vi "更新程序.vi"() -> ()   [LabVIEW 2016, in "自动更新.lvlib"]
uses:
  <vilib>/FTP/NI_FTP.lvlib
panel:
  out "FTP链接结束":bool
  out "updateconfiguration":T1
  out "软件版本 2":string caption="目标软件版本"
  out "软件版本":string caption="当前软件版本"
  out "下载的文件名":string
  out "目标文件夹名":string
  out "端口号":i32
  out "IP地址":string
  out "步骤":string
  out "枚举":T2(ring)
  in  "目标路径（使用对话框）":path
  out "下载保存目录":path
  out "更新进度":u8(slide) scale=0.0..100.0
  # "1.先下载更新-------2.关闭主应用-------3.替换应用--------4.打开主应用-----------5.关闭本程序"
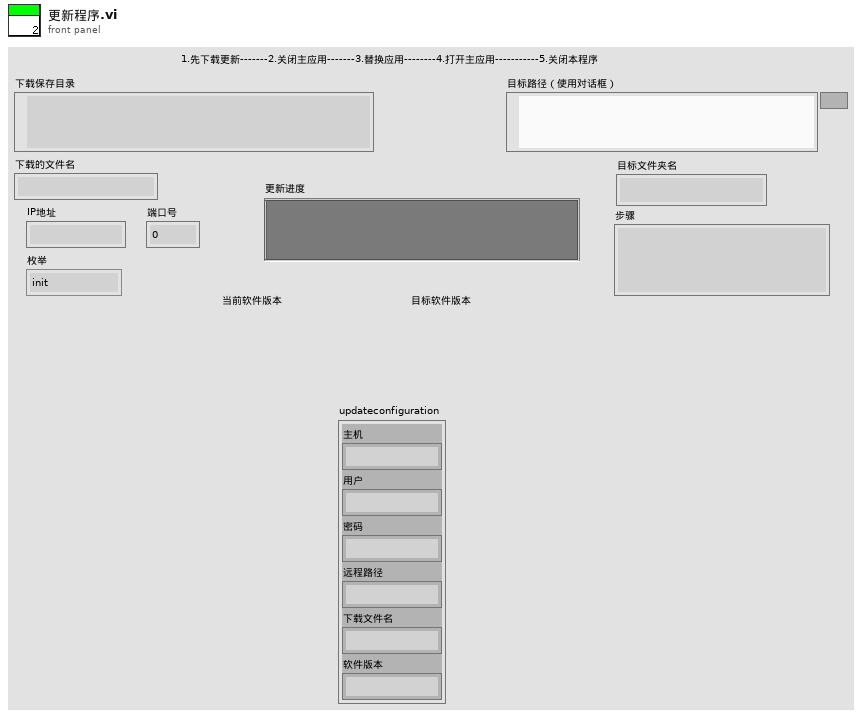
[diagram p1: front panel]
types:
  T1 = cluster{"主机":string, "用户":string, "密码":string, "远程路径":string, "下载文件名":string, "软件版本":string}
  T2 = enum16{"init", "download", "close", "replace", "open", "over"}
  T3 = typedef "NI_FTP.lvlib/FTP File Info.ctl" = cluster{"type":enum16{"unknown", "file", "dir", "link"}, "permissions":string, "owner":string, "group":string, "size":i32, "date":string, "name":string, "link name":string}
  T4 = enum16{"open", "replace", "create", "open or create", "replace or create", "replace or create with confirmation"}
  T5 = cluster{"网络灯":bool, "接收中":bool, "已接收百分比":u8, "接收成功次数":dbl, "当前步骤":enum16{"init", "receivehead", "receivecontent", "receivesuccess", "over"}, "文件名":string, "error out":errorcluster}
  T6 = cluster{"remote path":string, "local path":path, "binary":bool}
  T7 = typedef "NI_FTP.lvlib/FTP Session.ctl" = refnum<k5>
  T8 = cluster{"remote path":string, "local path":path, "binary":bool}[]
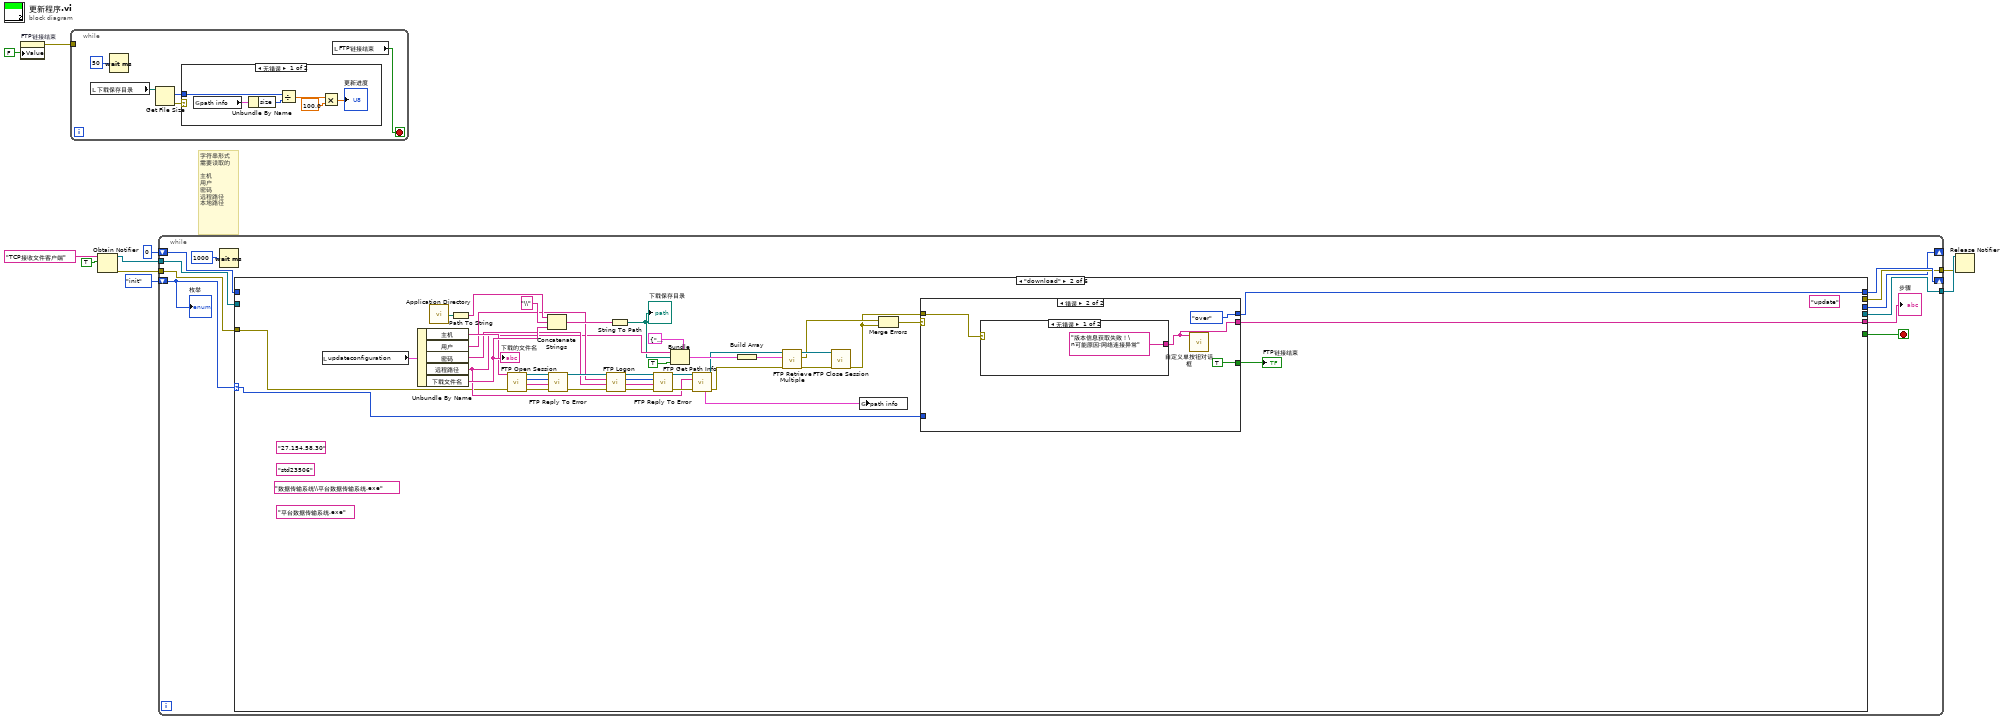
[diagram p0: block diagram]
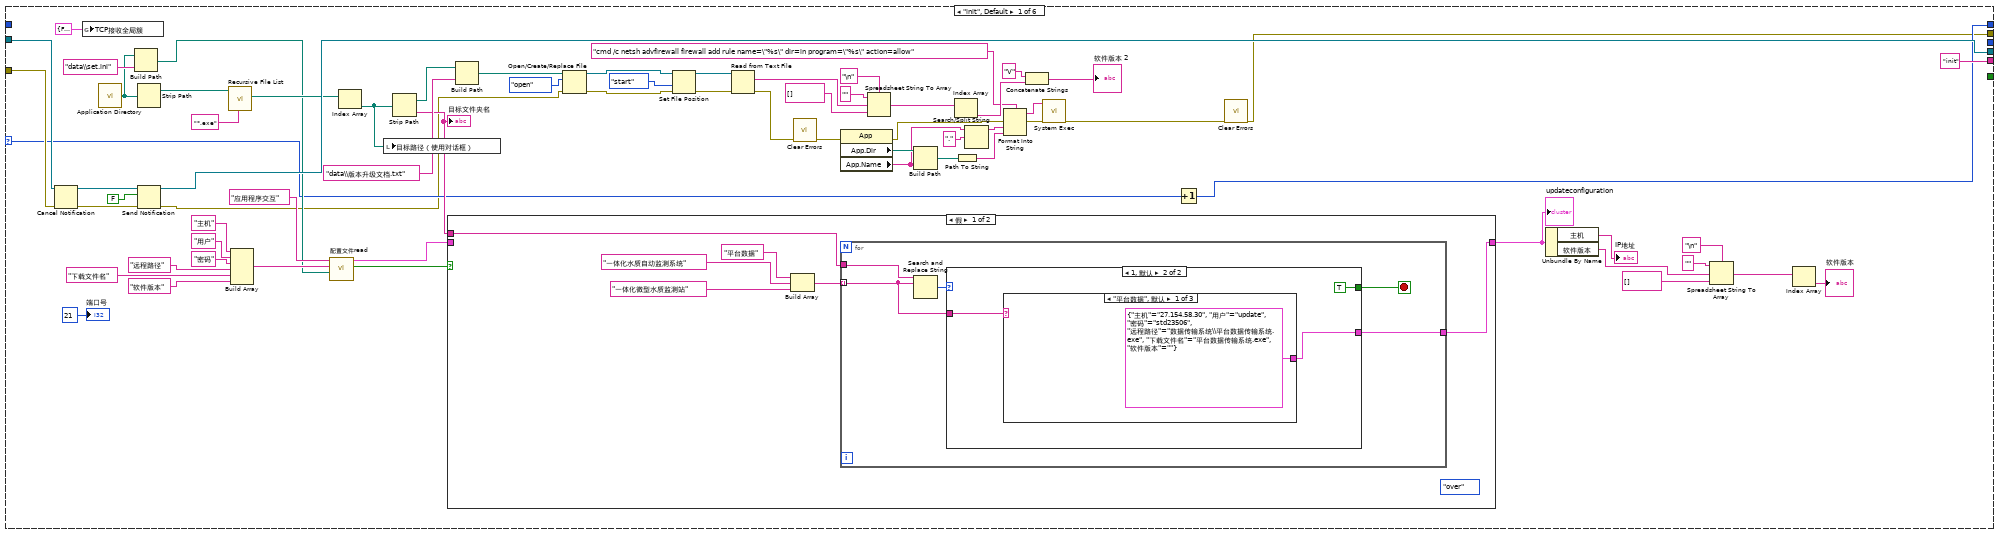
[diagram p3: hidden frame]
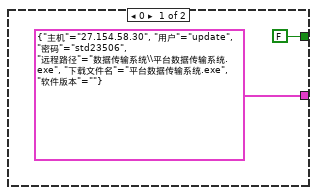
[diagram p4: hidden frame]
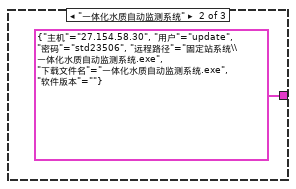
[diagram p5: hidden frame]
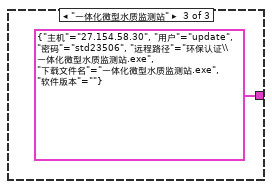
[diagram p6: hidden frame]
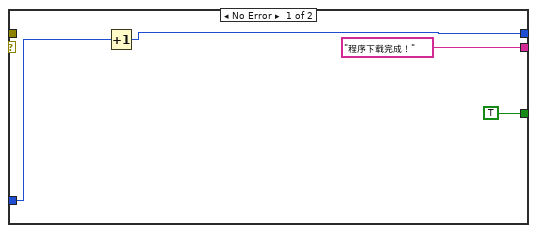
[diagram p8: hidden frame]
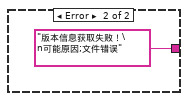
[diagram p9: hidden frame]
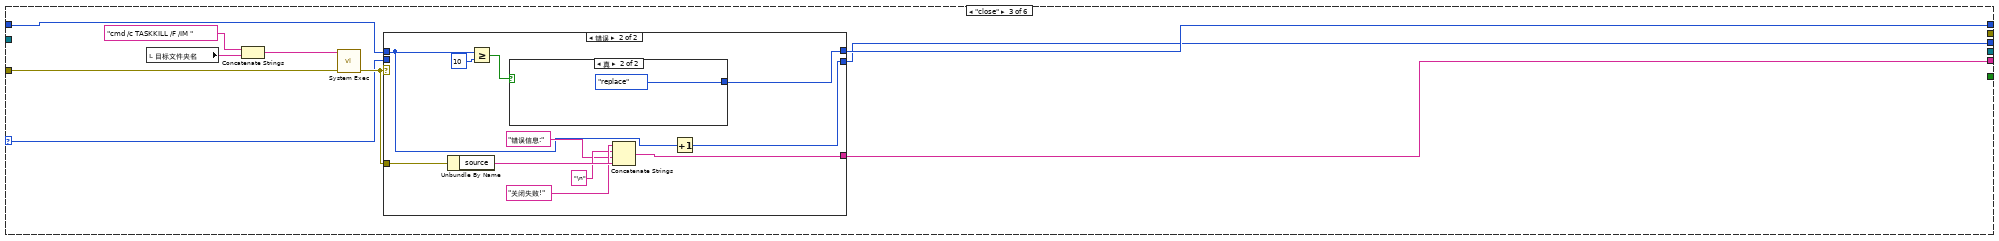
[diagram p10: hidden frame]
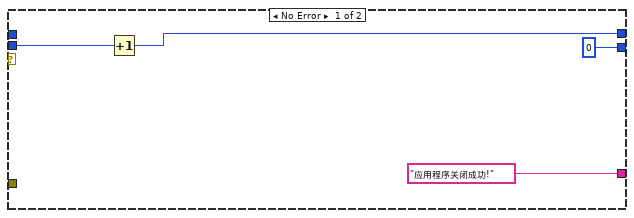
[diagram p11: hidden frame]
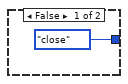
[diagram p12: hidden frame]
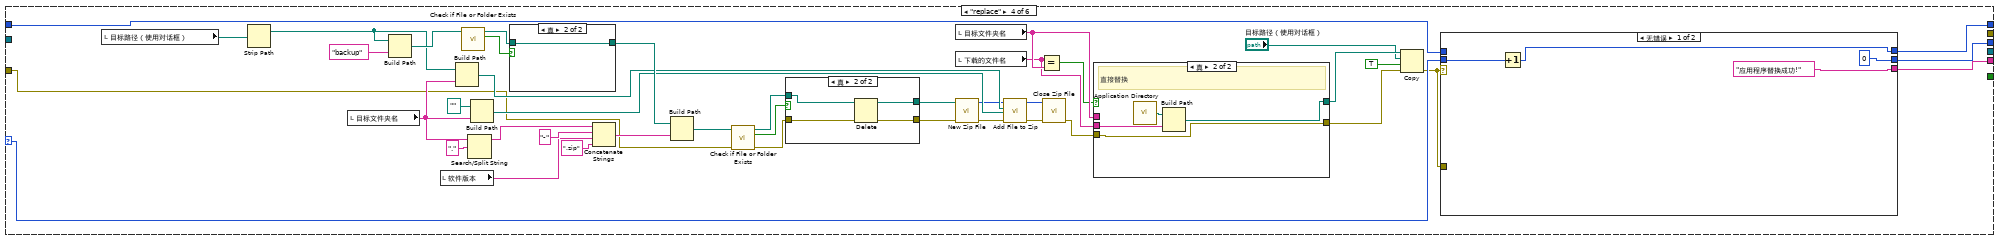
[diagram p13: hidden frame]
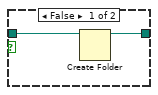
[diagram p15: hidden frame]
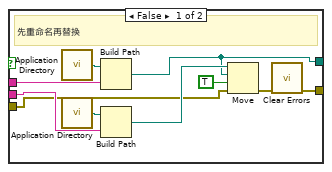
[diagram p16: hidden frame]
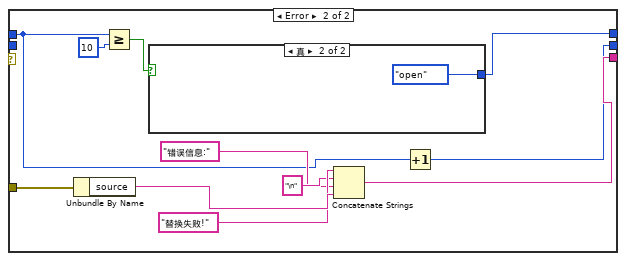
[diagram p17: hidden frame]
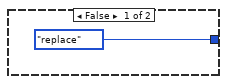
[diagram p18: hidden frame]
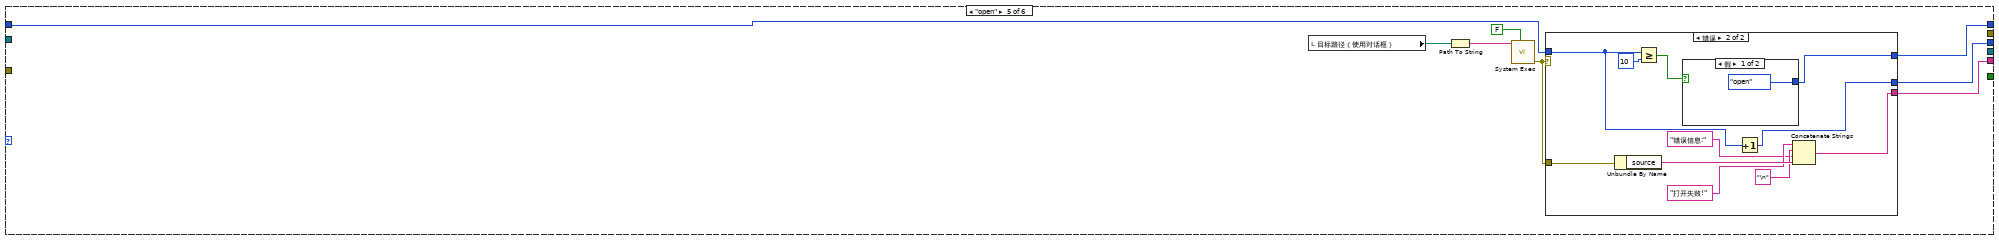
[diagram p19: hidden frame]
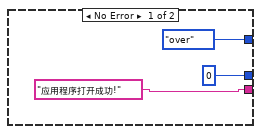
[diagram p20: hidden frame]
diagram:
  # "字符串形式\n需要读取的\n\n主机\n用户\n密码\n远程路径\n本地路径"
  n1 = property on="FTP链接结束" class="Bool (严格)"("Value"=FALSE ("FTP链接结束")) -> (error out=w1:errorcluster)  [unwired: 2 in, 1 out]
  n2 = while {
    tunnel: w1 -> [_]
    stop <- w15 stop-if-true
    n3 = local read "下载保存目录"() -> (w13:path)
    n4 = Wait (ms)(milliseconds to wait=u32 50 ("等待时间（毫秒）")) -> ()  [unwired: 1 out]
    n5 = Get File Size(file=w13) -> (size (in bytes)=w11:i64, 0:w12:errorcluster)  [unwired: 1 in, 1 out]
    n6 = case shown="无错误" w12 {
      tunnel: w11 -> [w17 _]
      frame No Error {
        n7 = global read "update全局.vi" "path info"() -> (w18:T3)
        n8 = Unbundle By Name(w18) -> ("size"=w21:i32)
        n9 = Divide(x=w17, y=w21) -> (x/y=w20:dbl)
        n10 = Multiply(x=w20, y=100.0) -> (x*y=→"更新进度":dbl)
      }
      frame Error {
      }
    }
    n11 = local read "FTP链接结束"() -> (w15:bool)
  }
  n12 = Obtain Notifier(name (unnamed)="TCP接收文件客户端" ("名称（未命名）"), notification data type=TRUE) -> (notifier out=w7:refnum<notifier>, error out=w6:errorcluster)  [unwired: 2 in, 1 out]
  n13 = while {
    shift-right: [w31] -> _
    shift-left: T2."init" -> [w32]
    tunnel: w7 -> [w27]
    tunnel: w6 -> [w26]
    tunnel: [w25] -> w5
    tunnel: [w24] -> w4
    shift-right: [w22] -> _
    shift-left: u8 0 -> [w23]
    stop <- w30 stop-if-true
    n14 = Wait (ms)(milliseconds to wait=u32 1000 ("等待时间（毫秒）")) -> ()  [unwired: 1 out]
    n15 = case shown="\"download\"" w32 {
      selector: w32 -> [w49 w159 w178 w240 _ w330]
      tunnel: [w48 w160 w177 w239 w284 w329] -> w31
      tunnel: [_ _ _ _ _ w325] -> w30
      tunnel: ["init" ("步骤") w158 w176 w238 w283 "over" ("步骤")] -> w28
      tunnel: w27 -> [w100 _ _ _ _ w327]
      tunnel: w26 -> [w99 w122 w172 w201 _ w305]
      tunnel: [w95 _ _ _ _ w326] -> w25
      tunnel: [w34 _ _ _ _ w310] -> w24
      tunnel: w23 -> [_ _ w174 w230 w281 _]
      tunnel: [_ _ w173 w229 w282 _] -> w22
      frame "init", Default {
        n16 = Cancel Notification(0:w100, 3:w99) -> (8:w98:refnum<notifier>, 11:w96:errorcluster)  [unwired: 1 out]
        n17 = global write "全局变量1.vi" "TCP接收全局簇"(T5 {"网络灯"=FALSE, "接收中"=FALSE, "已接收百分比"=0, "接收成功次数"=0.0, "当前步骤"=enum."init", "文件名"="", "error out"={"status"=FALSE, "code"=0, "source"=""}} ("TCP接收全局簇")) -> ()
        n18 = call <vilib>:"Application Directory.vi"() -> ("Application Directory"=w56:path)
        n19 = Build Path(base path=w56, name or relative path="data\\set.ini" ("名称或相对路径")) -> (appended path=w59:path)
        n20 = Strip Path(path=w56) -> (stripped path=w90:path)  [unwired: 1 out]
        n21 = Send Notification(notification=FALSE ("通知"), notifier=w98, error in (no error)=w96) -> (notifier out=w95:refnum<notifier>, error out=w35:errorcluster)
        n22 = call <vilib>:"Recursive File List.vi"("pattern"="*.exe", "Folder Path"=w90) -> ("All Files in Dir"=w92:path[])  [unwired: 5 in, 4 out]
        n23 = Build Array("主机" ("section"), "用户" ("section"), "密码" ("key"), "远程路径" ("key"), "下载文件名" ("key"), "软件版本" ("key")) -> (w63:string[])
        n24 = call "配置文件read.vi"("configuration file path"=w59, "键数组"=w63, "段"="应用程序交互" ("section")) -> ("section exists?"=w65:bool, "updateconfiguration"=w66:T1)  [unwired: 6 in, 1 out]
        n25 = Index Array(array=w92) -> (element=w93:path)  [unwired: 1 in]
        n26 = local write "目标路径（使用对话框）"(w93) -> ()
        n27 = Strip Path(path=w93) -> (stripped path=w67:path, name=w50:string)
        "目标文件夹名" <- w50
        n28 = case shown="假" w65 {
          tunnel: w66 -> [_ w121]
          tunnel: [w102 w121] -> w58
          tunnel: w50 -> [w103 _]
          frame False {
            (unwired) T2."over"
            n29 = Build Array("平台数据" ("搜索字符串"), "一体化水质自动监测系统" ("搜索字符串"), "一体化微型水质监测站" ("搜索字符串")) -> (w104:string[])
            n30 = for {
              tunnel: w104 -> [w109] mode=indexing
              tunnel: w103 -> [w110]
              tunnel: [w108] -> w102
              stop <- w111 stop-if-true
              n31 = Search and Replace String(input string=w110, search string=w109) -> (number of replacements=w112:i32)  [unwired: 6 in, 3 out]
              n32 = case shown="1, 默认" w112 {
                tunnel: [FALSE TRUE] -> w111
                tunnel: w109 -> [_ w116]
                tunnel: [T1 {"主机"="27.154.58.30", "用户"="update", "密码"="std23506", "远程路径"="数据传输系统\\平台数据传输系统.exe", "下载文件名"="平台数据传输系统.exe", "软件版本"=""} ("updateconfiguration") w115] -> w108
                frame 0 {
                }
                frame 1, Default {
                  n33 = case shown="\"平台数据\", 默认" w116 {
                    tunnel: [T1 {"主机"="27.154.58.30", "用户"="update", "密码"="std23506", "远程路径"="数据传输系统\\平台数据传输系统.exe", "下载文件名"="平台数据传输系统.exe", "软件版本"=""} ("updateconfiguration") T1 {"主机"="27.154.58.30", "用户"="update", "密码"="std23506", "远程路径"="固定站系统\\一体化水质自动监测系统.exe", "下载文件名"="一体化水质自动监测系统.exe", "软件版本"=""} ("updateconfiguration") T1 {"主机"="27.154.58.30", "用户"="update", "密码"="std23506", "远程路径"="环保认证\\一体化微型水质监测站.exe", "下载文件名"="一体化微型水质监测站.exe", "软件版本"=""} ("updateconfiguration")] -> w115
                    frame "平台数据", Default {
                    }
                    frame "一体化水质自动监测系统" {
                    }
                    frame "一体化微型水质监测站" {
                    }
                  }
                }
              }
            }
          }
          frame True {
          }
        }
        "updateconfiguration" <- w58
        n34 = Build Path(base path=w67, name or relative path="data\\版本升级文档.txt" ("名称或相对路径")) -> (appended path=w75:path)
        n35 = Open/Create/Replace File(file path (use dialog)=w75, error in=w35, operation (0:open)=T4."open" ("操作(0:open)")) -> (refnum out=w70:refnum<file>, error out=w71:errorcluster)  [unwired: 3 in, 1 out]
        n36 = Set File Position(refnum=w70, from (0:start)=enum16{"start", "end", "current"}."start" ("自（0:起始）"), error in=w71) -> (refnum out=w74:refnum<file>, error out=w72:errorcluster)  [unwired: 1 in]
        n37 = Read from Text File(file (use dialog)=w74, error in=w72) -> (text=w82:string, error out=w39:errorcluster)  [unwired: 2 in, 2 out]
        n38 = call <vilib>:"Clear Errors.vi"("error in (no error)"=w39) -> ("error out"=w33:errorcluster)  [unwired: 5 in, 1 out]
        n39 = property class="App"(error in=w33) -> (error out=w38:errorcluster, "App.Dir"=w47:path, "App.Name"=w42:string)  [unwired: 1 in, 1 out]
        n40 = Spreadsheet String To Array(delimiter (Tab)="\n" ("分隔符(Tab)"), format string="" ("格式字符串"), spreadsheet string=w82, array type (2D Dbl)=string[] []) -> (array=w79:string[])
        n41 = Build Path(base path=w47, name or relative path=w42) -> (appended path=w46:path)
        n42 = Index Array(array=w79) -> (element=w80:string)  [unwired: 1 in]
        n43 = Path To String(path=w46) -> (string=w44:string)
        n44 = Search/Split String(string=w42, search string/char (-)="." ("搜索字符串/字符(-)")) -> (substring before match=w41:string)  [unwired: 1 in, 2 out]
        n45 = Format Into String(format string="cmd /c netsh advfirewall firewall add rule name=\"%s\" dir=in program=\"%s\" action=allow" ("command line"), error in=w38, w41, w44) -> (resulting string=w40:string, error out=w37:errorcluster)  [unwired: 1 in]
        n46 = Concatenate Strings("V" ("字符串"), w80) -> (→"软件版本 2":string)
        n47 = call <vilib>:"System Exec.vi"("error in (no error)"=w37, "command line"=w40) -> ("error out"=w36:errorcluster)  [unwired: 6 in, 3 out]
        n48 = Increment(x=w49) -> (x+1=w48:T2)
        n49 = call <vilib>:"Clear Errors.vi"("error in (no error)"=w36) -> ("error out"=w34:errorcluster)  [unwired: 5 in, 1 out]
        n50 = Unbundle By Name(w58) -> ("主机"=→"IP地址":string, "软件版本"=w51:string)
        n51 = Spreadsheet String To Array(delimiter (Tab)="\n" ("分隔符(Tab)"), format string="" ("格式字符串"), spreadsheet string=w51, array type (2D Dbl)=string[] []) -> (array=w85:string[])
        n52 = Index Array(array=w85) -> (element=→"软件版本":string)  [unwired: 1 in]
        "端口号" <- 21 ("端口号")
      }
      frame "download" {
        (unwired) "平台数据传输系统.exe" ("字符串")
        (unwired) "std23506" ("password")
        (unwired) "update" ("user")
        (unwired) "数据传输系统\\平台数据传输系统.exe" ("remote path")
        (unwired) "27.154.58.30" ("host")
        n53 = local read "updateconfiguration"() -> (w154:T1)
        n54 = Unbundle By Name(w154) -> ("主机"=w139:string, "用户"=w138:string, "密码"=w137:string, "远程路径"=w134:string, "下载文件名"=w152:string)
        "下载的文件名" <- w152
        n55 = call <vilib>:"Application Directory.vi"() -> ("Application Directory"=w157:path)
        n56 = Path To String(path=w157) -> (string=w156:string)
        n57 = call <vilib>:"FTP Open Session.vi"("error in (no error)"=w122, "address"=w139) -> ("error out"=w141:errorcluster, "reply string"=w143:string, "reply code"=w142:i32, "ftp session"=w140:T7)  [unwired: 2 in, 4 out]
        n58 = Concatenate Strings(w156, "\\" ("字符串"), w152) -> (w155:string)
        n59 = call <vilib>:"FTP Reply To Error.vi"("error in (no error)"=w141, "reply string in"=w143, "reply code in"=w142, "ftp session"=w140) -> ("error out"=w144:errorcluster, "ftp session out"=w145:T7)  [unwired: 2 out]
        n60 = call <vilib>:"FTP Logon.vi"("error in (no error)"=w144, "password"=w137, "user"=w138, "ftp session"=w145) -> ("error out"=w146:errorcluster, "reply string"=w148:string, "reply code"=w149:i32, "ftp session out"=w147:T7)  [unwired: 4 out]
        n61 = String To Path(string=w155) -> (path=w133:path)
        "下载保存目录" <- w133
        n62 = call <vilib>:"FTP Reply To Error.vi"("error in (no error)"=w146, "reply string in"=w148, "reply code in"=w149, "ftp session"=w147) -> ("error out"=w151:errorcluster, "ftp session out"=w150:T7)  [unwired: 2 out]
        n63 = Bundle(cluster=T6 {"remote path"="", "local path"=path "", "binary"=FALSE} ("transfer spec"), "remote path"=w134, "local path"=w133, "binary"=TRUE) -> (w136:T6)
        n64 = call <vilib>:"FTP Get Path Info.vi"("error in (no error)"=w151, "remote path"=w134, "ftp session"=w150) -> ("error out"=w129:errorcluster, "ftp session out"=w131:T7, "path info"=w130:T3)  [unwired: 4 in, 2 out]
        n65 = Build Array(w136) -> (w128:T8)
        n66 = call <vilib>:"FTP Retrieve Multiple.vi"("error in (no error)"=w129, "file specifications"=w128, "ftp session"=w131) -> ("error out"=w126:errorcluster, "file errors"=w125:errorcluster[], "ftp session out"=w127:T7)  [unwired: 2 in, 4 out]
        n67 = call <vilib>:"FTP Close Session.vi"("error in (no error)"=w126, "ftp session"=w127) -> ("error out"=w124:errorcluster)  [unwired: 9 out]
        n68 = global write "update全局.vi" "path info"(w130) -> ()
        n69 = Merge Errors(w125, w124) -> (w161:errorcluster)
        n70 = case shown="错误" w161 {
          tunnel: w124 -> [_ w169]
          tunnel: [w165 T2."over"] -> w160
          tunnel: w159 -> [w164 _]
          tunnel: ["程序下载完成！" w167] -> w158
          tunnel: [TRUE ("FTP链接结束") TRUE ("FTP链接结束")] -> w123
          frame No Error {
            n71 = Increment(x=w164) -> (x+1=w165:T2)
          }
          frame Error {
            n72 = case shown="无错误" w169 {
              tunnel: ["版本信息获取失败！\n可能原因;网络连接异常" "版本信息获取失败！\n可能原因;文件错误"] -> w167
              frame No Error {
              }
              frame Error {
              }
            }
            n73 = call "自定义单按钮对话框.vi"("消息"=w167) -> ()  [unwired: 11 in]
          }
        }
        "FTP链接结束" <- w123
      }
      frame "close" {
        n74 = local read "目标文件夹名"() -> (w175:string)
        n75 = Concatenate Strings("cmd /c TASKKILL /F /IM " ("command line"), w175) -> (w179:string)
        n76 = call <vilib>:"System Exec.vi"("error in (no error)"=w172, "command line"=w179) -> ("error out"=w181:errorcluster)  [unwired: 6 in, 3 out]
        n77 = case shown="错误" w181 {
          tunnel: [w183 w190] -> w177
          tunnel: w181 -> [_ w196]
          tunnel: ["应用程序关闭成功!" ("步骤") w191] -> w176
          tunnel: w178 -> [w184 _]
          tunnel: w174 -> [_ w186]
          tunnel: [u8 0 w188] -> w173
          frame No Error {
            n78 = Increment(x=w184) -> (x+1=w183:T2)
          }
          frame Error {
            n79 = Unbundle By Name(w196) -> ("source"=w195:string)
            n80 = Greater Or Equal?(x=w186, y=u8 10) -> (x >= y?=w187:bool)
            n81 = case shown="真" w187 {
              tunnel: [T2."close" T2."replace"] -> w190
              frame False {
              }
              frame True {
              }
            }
            n82 = Concatenate Strings("关闭失败!" ("消息"), "\n" ("字符串"), "错误信息:" ("字符串"), w195) -> (w191:string)
            n83 = Increment(x=w186) -> (x+1=w188:u8)
          }
        }
      }
      frame "replace" {
        n84 = local read "目标路径（使用对话框）"() -> (w205:path)
        n85 = Strip Path(path=w205) -> (stripped path=w204:path)  [unwired: 1 out]
        n86 = local read "目标文件夹名"() -> (w203:string)
        n87 = Build Path(base path=w204, name or relative path="backup" ("名称或相对路径")) -> (appended path=w220:path)
        n88 = local read "软件版本"() -> (w206:string)
        n89 = Build Path(base path=w204, name or relative path=w203) -> (appended path=w217:path)
        n90 = call <vilib>:"Check if File or Folder Exists.vi"("path"=w220) -> ("file or folder exists?"=w221:bool, "dup path"=w222:path)  [unwired: 8 in, 1 out]
        n91 = Search/Split String(string=w203, search string/char (-)="." ("搜索字符串/字符(-)")) -> (substring before match=w211:string)  [unwired: 1 in, 2 out]
        n92 = Build Path(base path=path "" ("Relative Path from 1 to 2"), name or relative path=w203) -> (appended path=w219:path)
        n93 = case shown="真" w221 {
          tunnel: w222 -> [w248 w249]
          tunnel: [w247 w249] -> w223
          frame False {
            n94 = Create Folder(path (use dialog)=w248) -> (created path=w247:path)  [unwired: 2 in, 2 out]
          }
          frame True {
          }
        }
        n95 = Concatenate Strings(w211, "-" ("字符串"), w206, ".zip" ("字符串")) -> (w212:string)
        n96 = Build Path(base path=w223, name or relative path=w212) -> (appended path=w226:path)
        n97 = call <vilib>:"Check if File or Folder Exists.vi"("error in (no error)"=w201, "path"=w226) -> ("error out"=w200:errorcluster, "file or folder exists?"=w225:bool, "dup path"=w224:path)  [unwired: 7 in]
        n98 = case shown="真" w225 {
          tunnel: w224 -> [w242 w246]
          tunnel: [w242 w245] -> w227
          tunnel: w200 -> [w241 w244]
          tunnel: [w241 w243] -> w199
          frame False {
          }
          frame True {
            n99 = Delete(path (use dialog)=w246, error in=w244) -> (deleted path=w245:path, error out=w243:errorcluster)  [unwired: 3 in, 1 out]
          }
        }
        n100 = call <vilib>:"New Zip File.vi"("error in (no error)"=w199, "target"=w227) -> ("error out"=w213:errorcluster, "zip file out"=w214:i64)  [unwired: 1 in, 3 out]
        n101 = local read "目标文件夹名"() -> (w234:string)
        n102 = local read "下载的文件名"() -> (w233:string)
        n103 = call <vilib>:"Add File to Zip.vi"("error in (no error)"=w213, "destination path in zip"=w219, "source file path"=w217, "zip file in"=w214) -> ("error out"=w216:errorcluster, "zip file out"=w215:i64)  [unwired: 6 in]
        n104 = Equal?(x=w233, y=w234) -> (x = y?=w232:bool)
        n105 = call <vilib>:"Close Zip File.vi"("error in (no error)"=w216, "zip file in"=w215) -> ("error out"=w202:errorcluster)  [unwired: 5 in]
        n106 = case shown="真" w232 {
          tunnel: w233 -> [w256 w262]
          tunnel: w234 -> [w255 _]
          tunnel: [w254 w261] -> w237
          tunnel: [w251 w260] -> w228
          tunnel: w202 -> [w250 w260]
          frame False {
            # "先重命名再替换"
            n107 = call <vilib>:"Application Directory.vi"() -> ("Application Directory"=w258:path)
            n108 = call <vilib>:"Application Directory.vi"() -> ("Application Directory"=w257:path)
            n109 = Build Path(base path=w258, name or relative path=w255) -> (appended path=w254:path)
            n110 = Build Path(base path=w257, name or relative path=w256) -> (appended path=w259:path)
            n111 = Move(source path=w259, error in=w250, 9:TRUE ("覆盖(F)"), 10:w254) -> (error out=w252:errorcluster)  [unwired: 1 in, 2 out]
            n112 = call <vilib>:"Clear Errors.vi"("error in (no error)"=w252) -> ("error out"=w251:errorcluster)  [unwired: 5 in, 1 out]
          }
          frame True {
            # "直接替换"
            n113 = call <vilib>:"Application Directory.vi"() -> ("Application Directory"=w263:path)
            n114 = Build Path(base path=w263, name or relative path=w262) -> (appended path=w261:path)
          }
        }
        n115 = Copy(8:w228, 9:TRUE ("覆盖(F)"), 10:"目标路径（使用对话框）", 11:w237) -> (0:w231:errorcluster)  [unwired: 1 in, 2 out]
        n116 = case shown="无错误" w231 {
          tunnel: [w265 w272] -> w239
          tunnel: w231 -> [_ w278]
          tunnel: ["应用程序替换成功!" ("步骤") w273] -> w238
          tunnel: w240 -> [w266 _]
          tunnel: w230 -> [_ w270]
          tunnel: [u8 0 w268] -> w229
          frame No Error {
            n117 = Increment(x=w266) -> (x+1=w265:T2)
          }
          frame Error {
            n118 = Unbundle By Name(w278) -> ("source"=w277:string)
            n119 = Greater Or Equal?(x=w270, y=u8 10) -> (x >= y?=w269:bool)
            n120 = case shown="真" w269 {
              tunnel: [T2."replace" T2."open"] -> w272
              frame False {
              }
              frame True {
              }
            }
            n121 = Concatenate Strings("替换失败!" ("消息"), "\n" ("字符串"), "错误信息:" ("字符串"), w277) -> (w273:string)
            n122 = Increment(x=w270) -> (x+1=w268:u8)
          }
        }
      }
      frame "open" {
        n123 = local read "目标路径（使用对话框）"() -> (w285:path)
        n124 = Path To String(path=w285) -> (string=w288:string)
        n125 = call <vilib>:"System Exec.vi"("wait until completion? (T)"=FALSE, "command line"=w288) -> ("error out"=w286:errorcluster)  [unwired: 6 in, 3 out]
        n126 = case shown="错误" w286 {
          tunnel: [T2."over" w296] -> w284
          tunnel: w286 -> [_ w302]
          tunnel: ["应用程序打开成功!" ("步骤") w297] -> w283
          tunnel: w281 -> [_ w294]
          tunnel: [u8 0 w292] -> w282
          frame No Error {
          }
          frame Error {
            n127 = Unbundle By Name(w302) -> ("source"=w301:string)
            n128 = Greater Or Equal?(x=w294, y=u8 10) -> (x >= y?=w293:bool)
            n129 = case shown="假" w293 {
              tunnel: [T2."open" T2."over"] -> w296
              frame False {
              }
              frame True {
              }
            }
            n130 = Increment(x=w294) -> (x+1=w292:u8)
            n131 = Concatenate Strings("打开失败!" ("消息"), "\n" ("字符串"), "错误信息:" ("字符串"), w301) -> (w297:string)
          }
        }
      }
      frame "over" {
        w325 = TRUE
        n132 = local read "软件版本 2"() -> (w307:string)
        n133 = local read "软件版本"() -> (w309:string)
        n134 = Concatenate Strings("更新完成！\n更新前版本号:" ("字符串"), w309, "\r", "更新后版本号:", w307, "\r") -> (w323:string)
        n135 = Build Array(w323) -> (w322:string[])
        n136 = call <vilib>:"Application Directory.vi"() -> ("Application Directory"=w320:path)
        n137 = call "更新log记录.vi"("路径"=w320, "错误输入（无错误）"=w305, "logname"="版本更新log", "数组"=w322) -> ("错误输出"=w318:errorcluster)  [unwired: 7 in]
        n138 = call <vilib>:"Clear Errors.vi"("error in (no error)"=w318) -> ("error out"=w317:errorcluster)  [unwired: 5 in, 1 out]
        n139 = Increment(x=w330) -> (x+1=w329:T2)
        n140 = Send Notification(notification=w325, notifier=w327, error in (no error)=w317) -> (notifier out=w326:refnum<notifier>, error out=w313:errorcluster)
        n141 = Current VI's Path() -> (path=w315:path)
        n142 = Open VI Reference(vi path=w315, error in (no error)=w313) -> (vi reference=w314:refnum<vi>, error out=w316:errorcluster)  [unwired: 4 in]
        n143 = invoke class="VI" method="FP.Close"(reference=w314, error in=w316) -> (reference out=w311:refnum<vi>, error out=w312:errorcluster)  [unwired: 1 in, 1 out]
        n144 = Close Reference(reference=w311, error in (no error)=w312) -> (error out=w310:errorcluster)
      }
    }
    "步骤" <- w28
    "枚举" <- w32
  }
  n145 = Release Notifier(notifier=w5, error in (no error)=w4) -> ()  [unwired: 1 in, 3 out]
